vi "Collect Average Measurement.vi"(8 "error in (no error)":errorcluster, 9 "Measurement Time[s]":dbl=0.5 format="%#_13g", 10 "channel name":string, 11 "UTP IO Session in":T1) -> (0 "error out":errorcluster, 1 "Values":dbl[](array[numeric]), 2 "Averaged value":dbl, 3 "UTP IO Session out":T1)   [LabVIEW 2023]
doc: "Collects single samples and calculates average value"
uses:
  <vilib>/Noffz/UTP IO/UTP IO Library/Typedefs/Session Handle.ctl
  <vilib>/Noffz/UTP IO/UTP IO Library/UTP IO Pool Session.lvclass
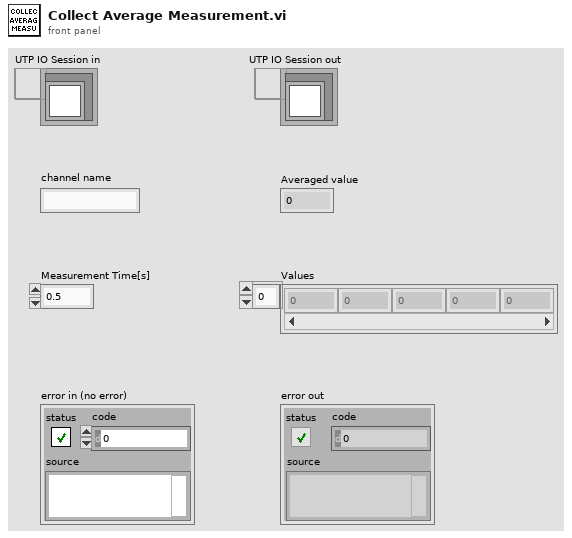
[diagram p1: front panel]
types:
  T1 = typedef "UTP IO Library.lvlib/UTP IO Pool Session.lvclass/Session Handle.ctl" = refnum<data-value>
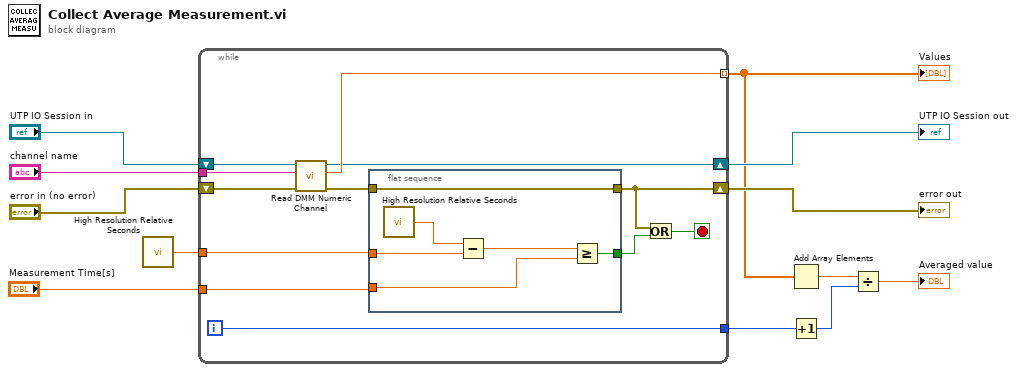
[diagram p0: block diagram]
diagram:
  n1 = call <vilib>:"High Resolution Relative Seconds.vi"() -> ("relative seconds"=w8:dbl)
  n2 = while {
    tunnel: "channel name" -> [w23]
    shift-right: [w18] -> w11
    shift-left: "UTP IO Session in" -> [w24]
    tunnel: w8 -> [w21]
    tunnel: [w20] -> w6 mode=indexing
    shift-right: [w15] -> w7
    shift-left: "error in (no error)" -> [w22]
    tunnel: [w17] -> w5
    tunnel: "Measurement Time[s]" -> [w16]
    i -> [w17]
    stop <- w13 stop-if-true
    n3 = call <vilib>:"Read DMM Numeric Channel.vi"("error in (no error)"=w22, "channel name"=w23, "UTP IO Session in"=w24) -> ("error out"=w19:errorcluster, "value"=w20:dbl, "UTP IO Session out"=w18:T1)  [unwired: 6 in]
    n4 = flat-sequence {
      tunnel: w21 -> [w30]
      tunnel: [w25] -> _
      tunnel: w19 -> [w28]
      tunnel: [w28] -> w15
      tunnel: w16 -> [w26]
      tunnel: [w25] -> w14
      frame #0 {
        n5 = call <vilib>:"High Resolution Relative Seconds.vi"() -> ("relative seconds"=w27:dbl)
        n6 = Subtract(x=w27, y=w30) -> (x-y=w29:dbl)
        n7 = Greater Or Equal?(x=w29, y=w26) -> (x >= y?=w25:bool)
      }
    }
    n8 = Or(x=w15, y=w14) -> (x .or. y?=w13:bool)
  }
  "UTP IO Session out" <- w11
  "Values" <- w6
  "error out" <- w7
  n9 = Add Array Elements(numeric array=w6) -> (sum=w4:dbl)
  n10 = Increment(x=w5) -> (x+1=w3:i32)
  n11 = Divide(x=w4, y=w3) -> (x/y=→"Averaged value":dbl)
